vi "Initialize.vi"(8 "error in (no error)":errorcluster, 10 "Connection String":string, 11 "MicronServer in":refnum<class "Server.lvclass">) -> (0 "error out":errorcluster, 2 "MessageUserEvent":refnum<user-event>, 3 "MicronServer out":refnum<class "Server.lvclass">)   [LabVIEW 2019, in "Micron.lvlib" / "Server.lvclass"]
uses:
  Server.lvclass
  Message/Message.lvclass
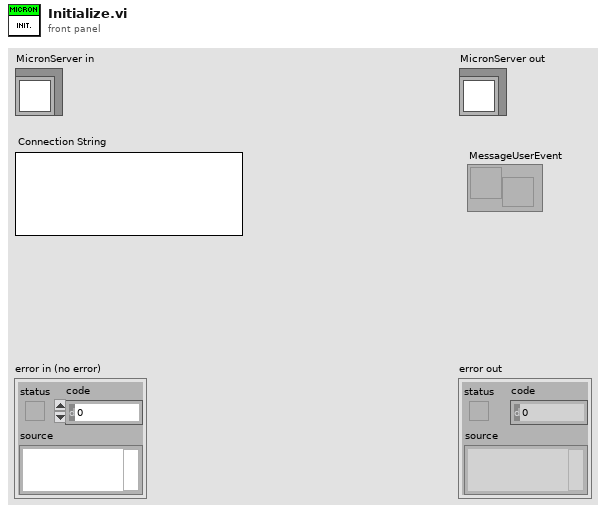
[diagram p1: front panel]
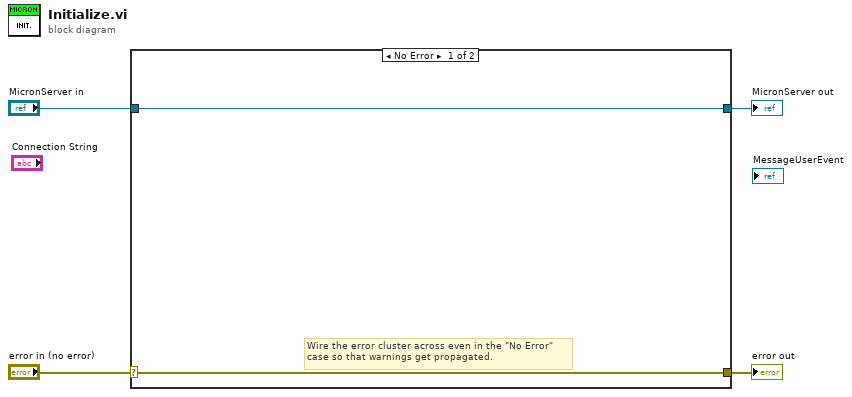
[diagram p0: block diagram]
diagram:
  n1 = case shown="No Error" "error in (no error)" {
    selector: "error in (no error)" -> [w5 w8]
    tunnel: [w5 w8] -> w3
    tunnel: [w6 w7] -> w1
    tunnel: "MicronServer in" -> [w6 w7]
    frame No Error {
      # "Wire the error cluster across even in the \"No Error\"\ncase so that warnings get propagated."
    }
    frame Error {
    }
  }
  "error out" <- w3
  "MicronServer out" <- w1
